vi "409b_TableMode.vi"(5 "Dwell (Hex)":string, 6 "Port":refnum<visa-resource-name>="COM1", 7 "Voltage":dbl, 8 "Phase":dbl, 9 "Frequency (MHz)":dbl, 10 "Memory (Hex)":string, 11 "Channel":u16(ring) items=["Ch0", "Ch1"]) -> (1 "Confirm":string, 2 "Response":string, 3 "Command":string)   [LabVIEW 2013]
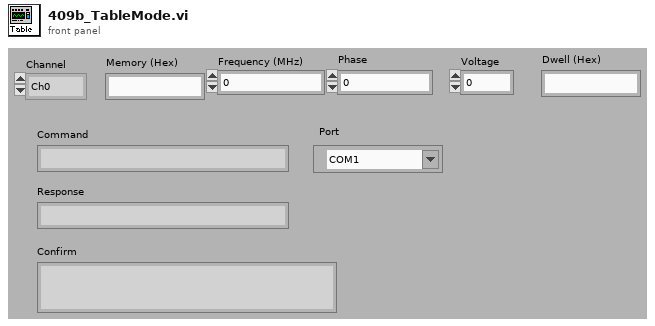
[diagram p1: front panel]
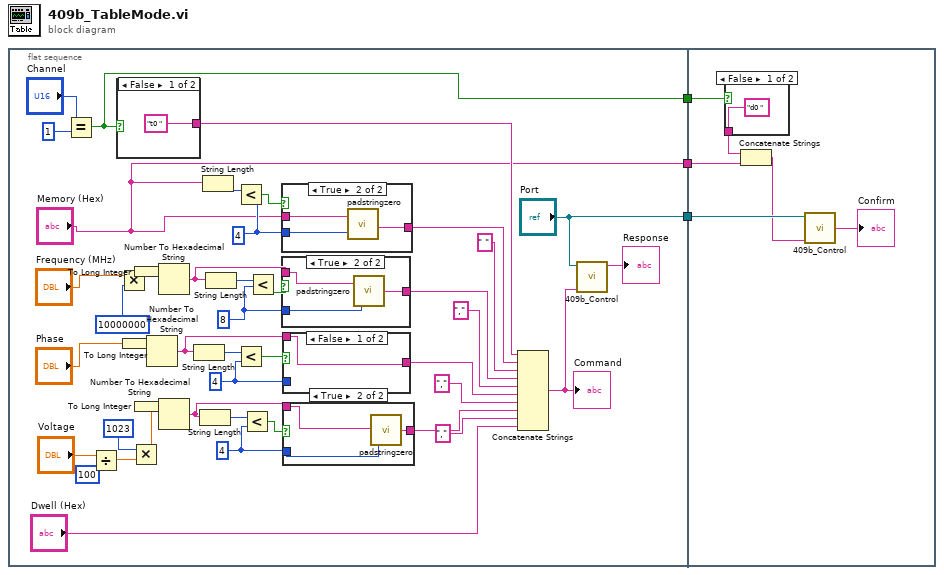
[diagram p0: block diagram]
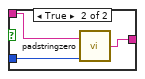
[diagram p3: hidden frame]
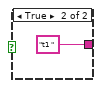
[diagram p6: hidden frame]
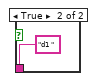
[diagram p7: hidden frame]
diagram:
  n1 = flat-sequence {
    tunnel: [w11] -> w3
    tunnel: ["Port"] -> w2
    tunnel: ["Memory (Hex)"] -> w1
    tunnel: w3 -> [w71]
    tunnel: w2 -> [w69]
    tunnel: w1 -> [w67]
    frame #0 {
      w29 = 4
      w16 = 4
      w22 = 4
      w25 = 8
      n2 = Equal?(x="Channel", y=1) -> (x = y?=w11:bool)
      n3 = Divide(x="Voltage", y=100) -> (x/y=w44:dbl)
      n4 = case shown="False" w11 {
        tunnel: ["t0 " "t1 "] -> w40
        frame False {
        }
        frame True {
        }
      }
      n5 = Multiply(x="Frequency (MHz)", y=10000000) -> (x*y=w26:dbl)
      n6 = To Long Integer(number="Phase") -> (32bit integer=w5:i32)
      n7 = To Long Integer(number=w26) -> (32bit integer=w4:i32)
      n8 = Multiply(x=1023, y=w44) -> (x*y=w15:dbl)
      n9 = To Long Integer(number=w15) -> (32bit integer=w6:i32)
      n10 = Number To Hexadecimal String(2:w5) -> (0:w21:string)  [unwired: 1 in]
      n11 = Number To Hexadecimal String(2:w4) -> (0:w24:string)  [unwired: 1 in]
      n12 = Number To Hexadecimal String(2:w6) -> (0:w14:string)  [unwired: 1 in]
      n13 = String Length(string=w21) -> (length=w23:i32)
      n14 = String Length(string=w14) -> (length=w17:i32)
      n15 = String Length(string="Memory (Hex)") -> (length=w30:i32)
      n16 = String Length(string=w24) -> (length=w28:i32)
      n17 = Less?(x=w30, y=w29) -> (x < y?=w31:bool)
      n18 = Less?(x=w23, y=w22) -> (x < y?=w19:bool)
      n19 = Less?(x=w17, y=w16) -> (x < y?=w18:bool)
      n20 = Less?(x=w28, y=w25) -> (x < y?=w27:bool)
      n21 = case shown="True" w31 {
        tunnel: "Memory (Hex)" -> [w60 w63]
        tunnel: [w60 w62] -> w32
        tunnel: w29 -> [_ w61]
        frame False {
        }
        frame True {
          n22 = call "padstringzero.vi"("Length"=w61, "str"=w63) -> ("res"=w62:string)
        }
      }
      n23 = case shown="True" w27 {
        tunnel: w25 -> [_ w59]
        tunnel: [w56 w58] -> w38
        tunnel: w24 -> [w56 w57]
        frame False {
        }
        frame True {
          n24 = call "padstringzero.vi"("Length"=w59, "str"=w57) -> ("res"=w58:string)
        }
      }
      n25 = case shown="False" w19 {
        tunnel: w22 -> [_ w55]
        tunnel: [w52 w54] -> w36
        tunnel: w21 -> [w52 w53]
        frame False {
        }
        frame True {
          n26 = call "padstringzero.vi"("Length"=w55, "str"=w53) -> ("res"=w54:string)
        }
      }
      n27 = case shown="True" w18 {
        tunnel: w16 -> [_ w51]
        tunnel: [w48 w50] -> w35
        tunnel: w14 -> [w48 w49]
        frame False {
        }
        frame True {
          n28 = call "padstringzero.vi"("Length"=w51, "str"=w49) -> ("res"=w50:string)
        }
      }
      n29 = Concatenate Strings(w40, w32, " ", w38, ",", w36, ",", w35, ",", "Dwell (Hex)") -> (w13:string)
      "Command" <- w13
      n30 = call "409b_Control.vi"("Port"="Port", "Command"=w13) -> ("Response"=→"Response":string)  [unwired: 8 in]
    }
    frame #1 {
      n31 = case shown="False" w71 {
        tunnel: ["d0 " "d1 "] -> w70
        frame False {
        }
        frame True {
        }
      }
      n32 = Concatenate Strings(w70, w67) -> (w68:string)
      n33 = call "409b_Control.vi"("Port"=w69, "Command"=w68) -> ("Response"=→"Confirm":string)  [unwired: 8 in]
    }
  }
